vi "create Behaviour.vi"(8 "error in (no error)":errorcluster caption="Fehler (Eingang, kein Fehler)", 11 "Burst Eingang":refnum<class "Burst.lvclass"> caption="DNL_LabVIEW Object in") -> (0 "error out":errorcluster caption="Fehler (Ausgang)", 1 "regex":string[](array[string]), 2 "response":bool[](array[boolean]), 3 "Burst Ausgang":refnum<class "Burst.lvclass"> caption="DNL_LabVIEW Object out")   [LabVIEW 2013, in "Burst.lvclass"]
uses:
  Burst.lvclass
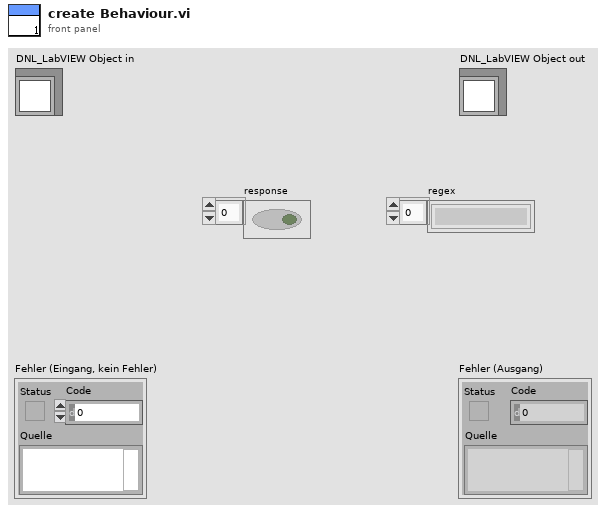
[diagram p1: front panel]
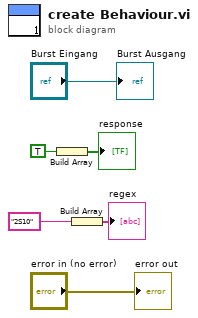
[diagram p0: block diagram]
diagram:
  n1 = Build Array(TRUE) -> (→"response":bool[])
  n2 = Build Array("2S10") -> (→"regex":string[])
  "error out" <- "error in (no error)"
  "Burst Ausgang" <- "Burst Eingang"
